vi "Correction_Logic_subvi.vi"(6 "Cluster":T1, 7 "FWHMx::1":dbl, 9 "MaxCounts::1":dbl, 10 "Target.X::1":dbl, 11 "centroidx::1":dbl) -> (1 "Max counts in range?":bool, 2 "Correction will be performed":bool, 3 "offset":dbl, 4 "FWHMx in range?":bool)   [LabVIEW 2013]
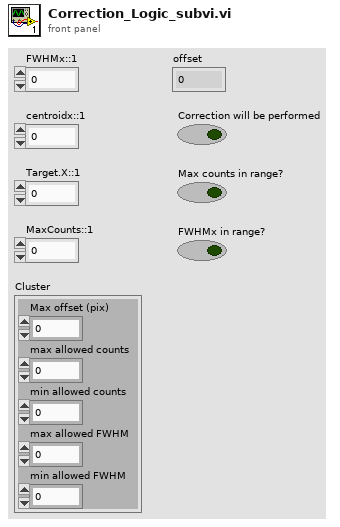
[diagram p1: front panel]
types:
  T1 = cluster{"Max offset (pix)":dbl, "max allowed counts":dbl, "min allowed counts":dbl, "max allowed FWHM":dbl, "min allowed FWHM":dbl}
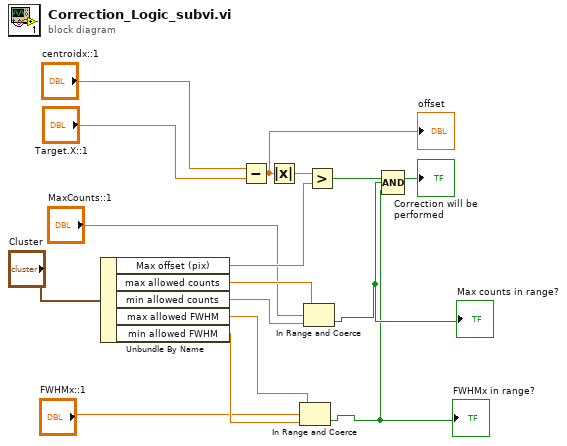
[diagram p0: block diagram]
diagram:
  n1 = Unbundle By Name("Cluster") -> ("Max offset (pix)"=w12:dbl, "max allowed counts"=w13:dbl, "min allowed counts"=w14:dbl, "max allowed FWHM"=w15:dbl, "min allowed FWHM"=w16:dbl)
  n2 = Subtract(x="centroidx::1", y="Target.X::1") -> (x-y=w6:dbl)
  "offset" <- w6
  n3 = Absolute Value(x=w6) -> (abs(x)=w5:dbl)
  n4 = In Range and Coerce(upper limit=w15, x="FWHMx::1", lower limit=w16) -> (In Range?=w1:bool)  [unwired: 1 out]
  "FWHMx in range?" <- w1
  n5 = In Range and Coerce(upper limit=w13, x="MaxCounts::1", lower limit=w14) -> (In Range?=w2:bool)  [unwired: 1 out]
  "Max counts in range?" <- w2
  n6 = Greater?(x=w5, y=w12) -> (0:w8:bool)
  n7 = Compound Arithmetic op=AND(w8, w2, w1) -> (→"Correction will be performed":bool)
